vi "parseStatus.vi"(8 "error in (no error)":errorcluster, 10 "response":string, 11 "XMLResponseParser In":refnum<class "XMLResponseParser.lvclass">) -> (0 "error out":errorcluster, 2 "status":string, 3 "XMLResponseParser Out":refnum<class "XMLResponseParser.lvclass">)   [LabVIEW 2023, in "AbstractFactory.lvlib" / "XMLResponseParser.lvclass"]
uses:
  XMLResponseParser.lvclass
  <vilib>/xml/Close Reference(Node).vi
  XMLResponseParser.lvclass/XMLResponseParser.ctl
  <vilib>/xml/NI_XML.lvlib
  <resource>/objmgr/DOMUserDefRef.rc
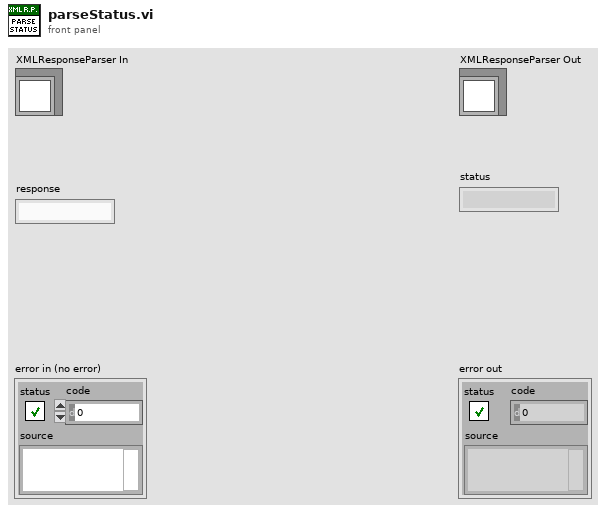
[diagram p1: front panel]
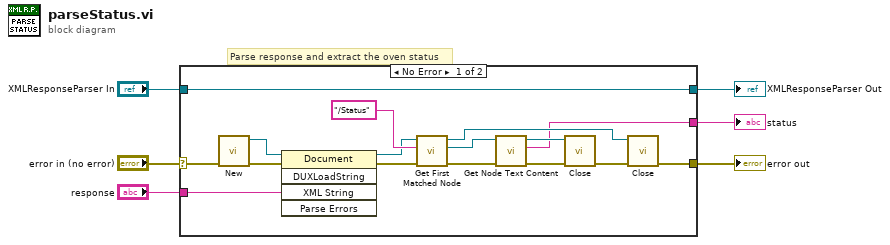
[diagram p0: block diagram]
diagram:
  # "Parse response and extract the oven status"
  n1 = case shown="No Error" "error in (no error)" {
    selector: "error in (no error)" -> [w19 w24]
    tunnel: [w13 w24] -> w5
    tunnel: [w8 w23] -> w3
    tunnel: "response" -> [w21 _]
    tunnel: "XMLResponseParser In" -> [w8 w23]
    tunnel: [w7 _] -> w1
    frame No Error {
      n2 = call <vilib>:"New.vi"("error in (no error)"=w19) -> ("error out"=w20:errorcluster, "DOM document out"=w22:refnum<k20>)  [unwired: 7 in]
      n3 = invoke class="Document" method="DUXLoadString"(reference=w22, error in=w20, "XML String"=w21) -> (reference out=w16:refnum<k20>, error out=w18:errorcluster)  [unwired: 2 in, 3 out]
      n4 = call <vilib>:"Get First Matched Node.vi"("error in (no error)"=w18, "XPath expression"="/Status", "node in"=w16) -> ("error out"=w12:errorcluster, "node result"=w10:refnum<k20>, "node out"=w14:refnum<k20>)  [unwired: 6 in]
      n5 = call <vilib>:"Get Node Text Content.vi"("error in (no error)"=w12, "node in"=w10) -> ("error out"=w11:errorcluster, "node text"=w7:string, "node out"=w9:refnum<k20>)  [unwired: 7 in]
      n6 = call-poly <vilib>:"Close.vi"("error in (no error)"=w11, "node"=w9) -> ("error out"=w15:errorcluster)  [unwired: 7 in]
      n7 = call-poly <vilib>:"Close.vi"("error in (no error)"=w15, "node"=w14) -> ("error out"=w13:errorcluster)  [unwired: 7 in]
    }
    frame Error {
    }
  }
  "error out" <- w5
  "XMLResponseParser Out" <- w3
  "status" <- w1
